vi "Get System Image.vi"   [LabVIEW 2017, in "nisyscfg.lvlib"]
doc: "<B>NOTE:</B> This VI has been replaced by the Create System Image VI on the Software Management palette.\n\nCreates a system image file or folder—a copy of the file contents on a primary hard drive of a system. The image can later be applied to a system to restore it to the state captured on the image."
uses:
  <vilib>/nisyscfg/nisyscfg.lvlib
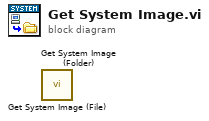
[diagram p0: block diagram]
diagram:
  n1 = call <vilib>:"Get System Image (File).vi"() -> ()  [unwired: 10 in, 2 out]
  n2 = call <vilib>:"Get System Image (Folder).vi"() -> ()  [unwired: 10 in, 2 out]
